vi "Test_WriteValue_InvalidType_Error.vi"(8 "error in (no error)":errorcluster, 11 "TestCase in":refnum<class "TestConfigurationFileBinding.lvclass">) -> (0 "error out":errorcluster, 3 "TestCase out":refnum<class "TestConfigurationFileBinding.lvclass">)   [LabVIEW 2017, in "TestConfigurationFileBinding.lvclass"]
uses:
  TestConfigurationFileBinding.lvclass
  TestConfigurationFileBinding.lvclass/TestConfigurationFileBinding.ctl
  Source/Concrete/ConfigurationFileBinding/ConfigurationFileBinding.lvclass/ConfigurationFileBinding.ctl
  Source/Concrete/ConfigurationFileBinding/ConfigurationFileBinding.lvclass
  C:/Git/composed-transport/Source/ITransport/ITransport.lvclass
  <vilib>/Utility/error.llb/Error Cluster From Error Code.vi
  <vilib>/Utility/config.llb/Not A Config Data Refnum.vi
  Source/ITransport/ITransport.lvclass
  <vilib>/Utility/config.llb/NI_LVConfig.lvlib
panel:
  out "Return Error":errorcluster
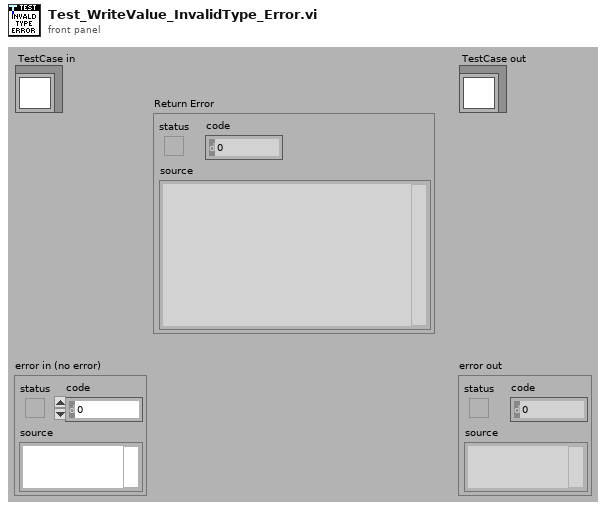
[diagram p1: front panel]
types:
  T1 = typedef "NI_LVConfig.lvlib/Config Data RefNum.ctl" = refnum<k1>
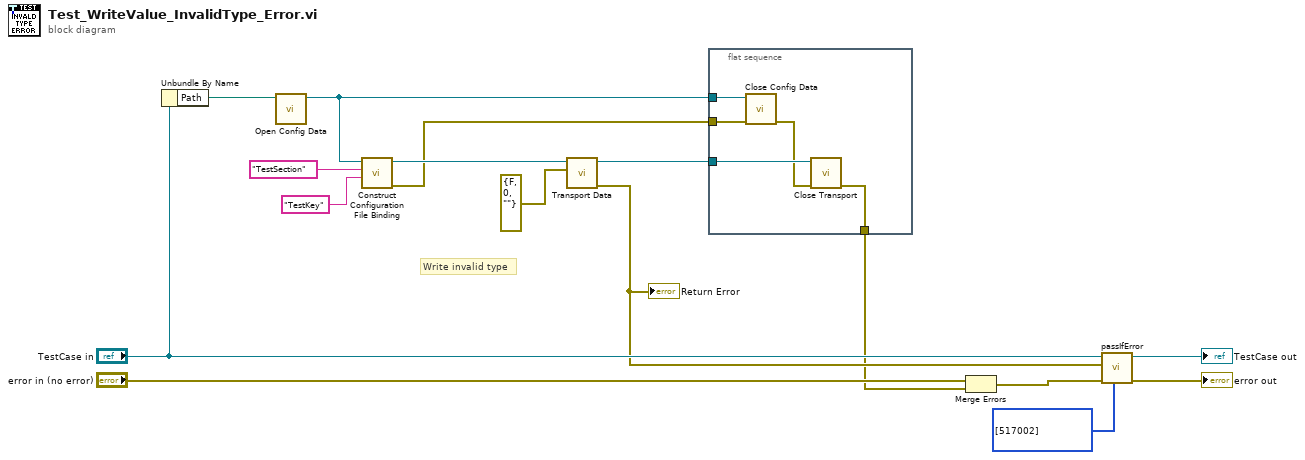
[diagram p0: block diagram]
diagram:
  # "Write invalid type"
  n1 = Unbundle By Name("TestCase in") -> ("Path"=w5:path)
  n2 = call <vilib>:"Open Config Data.vi"("configuration file path"=w5) -> ("refnum"=w11:T1)  [unwired: 8 in, 2 out]
  n3 = call "Construct Configuration File Binding.vi"("Key Name"="TestKey", "Section Name"="TestSection", "Config File Refnum"=w11) -> ("error out"=w4:errorcluster, "ConfigurationFileBinding"=w8:refnum<class "ConfigurationFileBinding.lvclass">)  [unwired: 7 in]
  n4 = call "Transport Data.vi"("Value"=errorcluster {"status"=FALSE, "code"=0, "source"=""} ("Test Value"), "ITransport in"=w8) -> ("error out"=w3:errorcluster, "ITransport out"=w16:refnum<class "ConfigurationFileBinding.lvclass">)  [unwired: 8 in]
  "Return Error" <- w3
  n5 = flat-sequence {
    tunnel: w16 -> [w21]
    tunnel: w11 -> [w19]
    tunnel: [w18] -> w2
    tunnel: w4 -> [w17]
    frame #0 {
      n6 = call <vilib>:"Close Config Data.vi"("error in (no error)"=w17, "refnum"=w19) -> ("error out"=w20:errorcluster)  [unwired: 8 in, 1 out]
      n7 = call-dynamic "Close Transport.vi"("error in (no error)"=w20, "ITransport in"=w21) -> ("error out"=w18:errorcluster)  [unwired: 9 in]
    }
  }
  n8 = Merge Errors("error in (no error)", w2) -> (w12:errorcluster)
  n9 = call-dynamic "passIfError.vi"("passing error codes (default = any error code)"=i32[] [517002], "error in (no error)"=w12, "error"=w3, "TestCase in"="TestCase in") -> ("error out"=→"error out":errorcluster, "TestCase out"=→"TestCase out":refnum<class "TestConfigurationFileBinding.lvclass">)  [unwired: 6 in]
